vi "Ingenjörsprojekt_Victor.vi"() -> ()   [LabVIEW 2020]
uses:
  <vilib>/DAQmx/read.llb/DAQmx Read (Analog Wfm 1Chan NSamp).vi
  <vilib>/DAQmx/miscellaneous.llb/DAQmx Fill In Error Info.vi
panel:
  out "Greatest from\nlatest sample":dbl
  in  "Clear Saved Data":bool
  in  "Path":path
  out "Graph 2 min":waveform(dbl)(graph)
  in  "Highest":dbl
  in  "Lowest":dbl
  in  "Alarm limit":dbl
  in  "Alarm toggle":bool
  out "Graph 30 min":waveform(dbl)(graph)
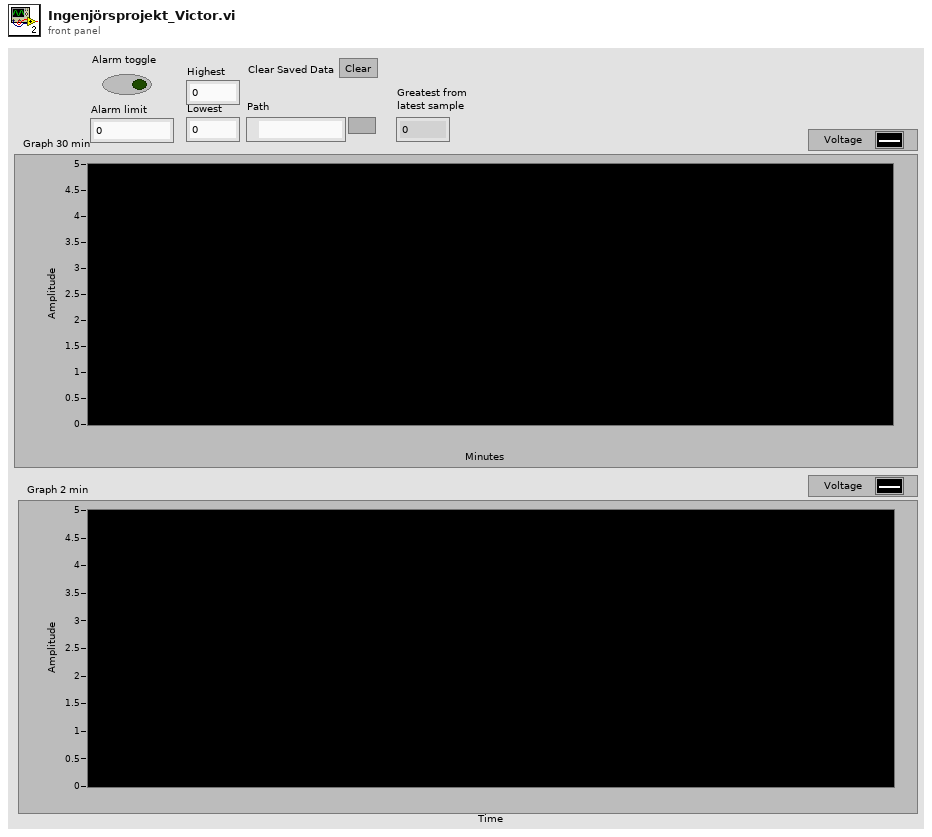
[diagram p1: front panel]
types:
  T1 = enum16{"open", "replace", "create", "open or create", "replace or create", "replace or create with confirmation"}
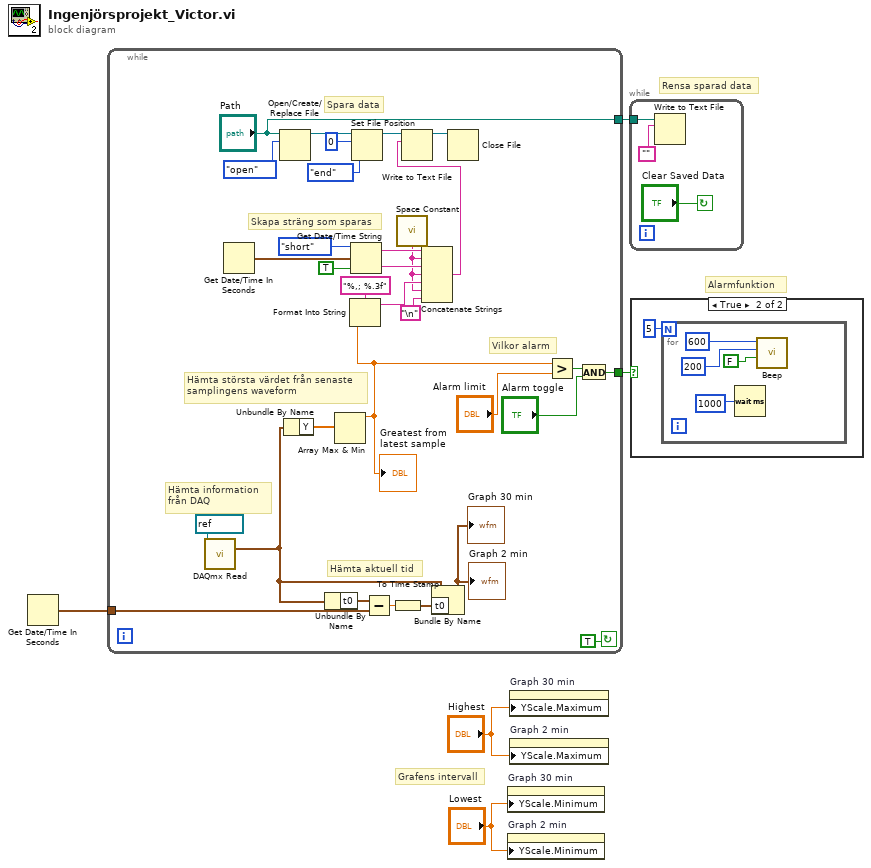
[diagram p0: block diagram]
diagram:
  # "Grafens intervall"
  # "Rensa sparad data"
  # "Alarmfunktion"
  n1 = Get Date/Time In Seconds() -> (seconds since 1Jan1904=w5:timestamp)
  n2 = while {
    tunnel: w5 -> [w27]
    tunnel: [w11] -> w2
    tunnel: ["Path"] -> w1
    stop <- TRUE continue-if-true
    # "Hämta aktuell tid"
    # "Hämta största värdet från senaste \nsamplingens waveform"
    # "Hämta information\nfrån DAQ"
    # "Vilkor alarm"
    # "Spara data"
    # "Skapa sträng som sparas"
    n3 = call-poly <vilib>:"DAQmx Read.vi"("task/channels in"=refnum<k21> "volt") -> ("data"=w10:waveform(dbl))  [unwired: 12 in, 2 out]
    n4 = Get Date/Time In Seconds() -> (seconds since 1Jan1904=w12:timestamp)
    n5 = Open/Create/Replace File(file path (use dialog)="Path", operation (0:open)=T1."open") -> (refnum out=w23:refnum<file>)  [unwired: 4 in, 2 out]
    n6 = Unbundle By Name(w10) -> ("Y"=w8:dbl[])
    n7 = Unbundle By Name(w10) -> ("t0"=w32:timestamp)
    n8 = Array Max & Min(array=w8) -> (max value=w6:dbl)  [unwired: 3 out]
    "Greatest from\nlatest sample" <- w6
    n9 = Format Into String(format string="%,; %.3f", w6) -> (resulting string=w15:string)  [unwired: 2 in, 1 out]
    n10 = Get Date/Time String(date format (0)=enum16{"short", "long", "abbreviated"}."short", seconds (now)=w12, want seconds? (F)=TRUE) -> (date string=w18:string, time string=w16:string)
    n11 = Set File Position(offset (in bytes) (0)=0, refnum=w23, from (0:start)=enum16{"start", "end", "current"}."end") -> (refnum out=w24:refnum<file>)  [unwired: 1 in, 1 out]
    n12 = Subtract(x=w32, y=w27) -> (x-y=w31:dbl)
    n13 = To Time Stamp(1:w31) -> (0:w30:timestamp)
    n14 = call <vilib>:"Space Constant.vi"() -> ("String"=w13:string)
    n15 = Concatenate Strings(w18, w13, w16, w13, w15, w13, "\n") -> (w9:string)
    n16 = Write to Text File(file (use dialog)=w24, text=w9) -> (refnum out=w21:refnum<file>)  [unwired: 2 in, 2 out]
    n17 = Bundle By Name(cluster=w10, "t0"=w30) -> (→"Graph 30 min" →"Graph 2 min":waveform(dbl))
    n18 = Close File(refnum=w21) -> ()  [unwired: 1 in, 2 out]
    n19 = Greater?(x=w6, y="Alarm limit") -> (0:w29:bool)
    n20 = And(x=w29, y="Alarm toggle") -> (x .and. y?=w11:bool)
  }
  n21 = property on="Graph 30 min" class="WFChart (strict)"("YScale.Minimum"="Lowest") -> ()  [unwired: 2 in, 2 out]
  n22 = property on="Graph 2 min" class="WFChart (strict)"("YScale.Minimum"="Lowest") -> ()  [unwired: 2 in, 2 out]
  n23 = property on="Graph 30 min" class="WFChart (strict)"("YScale.Maximum"="Highest") -> ()  [unwired: 2 in, 2 out]
  n24 = property on="Graph 2 min" class="WFChart (strict)"("YScale.Maximum"="Highest") -> ()  [unwired: 2 in, 2 out]
  n25 = while {
    tunnel: w1 -> [w37]
    stop <- "Clear Saved Data" continue-if-true
    n26 = Write to Text File(file (use dialog)=w37, text="") -> ()  [unwired: 2 in, 3 out]
  }
  n27 = case shown="True" w2 {
    frame False {
    }
    frame True {
      n28 = for {
        N: 5 -> [_]
        n29 = Wait (ms)(milliseconds to wait=1000) -> ()  [unwired: 1 out]
        n30 = call <vilib>:"Beep.vi"("use system alert? (T)"=FALSE, "duration (msec)"=200, "frequency (Hz)"=600) -> ()  [unwired: 9 in]
      }
    }
  }
